vi "3.vi"(11 "y":dbl) -> (3 "x+y":dbl)   [LabVIEW 2023]
panel:
  in  "x":dbl
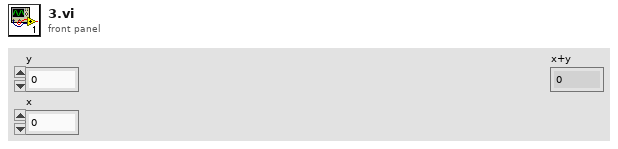
[diagram p1: front panel]
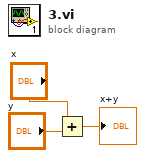
[diagram p0: block diagram]
diagram:
  n1 = Add(x="x", y="y") -> (x+y=→"x+y":dbl)
